vi "Configure FFT Measurement Trigger.vi"(4 "Trigger Timeout (1.0)":dbl=1.0 format="%^.3e", 5 "Offset (0.0)":dbl format="%^.3e", 6 "Threshold (-30.0)":dbl=-30.0 format="%^.3e", 7 "Slope (Rising)":i32(ring) items=["Rising", "Falling"], 8 "error in (no error)":errorcluster, 9 "Source (\"Free Run\")":string="Free Run", 10 "Instance (1)":i32=1, 11 "VISA resource name":refnum<visa-resource-name>) -> (0 "error out":errorcluster, 3 "VISA resource name out":refnum<visa-resource-name>)   [LabVIEW 2020, in "Rohde&Schwarz CMXP GPRF.lvlib"]
doc: "Defines the trigger parameters.\n\nAttributes:\nRSCMXPGPRF_ATTR_FFT_MEASUREMENT_TRIGGER_SOURCE\nRSCMXPGPRF_ATTR_FFT_MEASUREMENT_TRIGGER_SLOPE\nRSCMXPGPRF_ATTR_FFT_MEASUREMENT_TRIGGER_THRESHOLD\nRSCMXPGPRF_ATTR_FFT_MEASUREMENT_TRIGGER_OFFSET\nRSCMXPGPRF_ATTR_FFT_MEASUREMENT_TRIGGER_TIMEOUT\n\nRemote-control commands:\nTRIGger:GPRF:MEAS<i>:FFTSanalyzer:SOURce\nTRIGger:GPRF:MEAS<i>:FFTSanalyzer:SLOPe\nTRIGger:GPRF:MEAS<i>:FFTSanalyzer:THReshold\nTRIGger:GPRF:MEAS<i>:FFTSanalyzer:OFFSet\nTRIGger:GPRF:MEAS<i>:FFTSanalyzer:TOUT"
uses:
  <instrlib>/Rohde&Schwarz CMXP GPRF/Rohde&Schwarz CMXP GPRF.lvlib
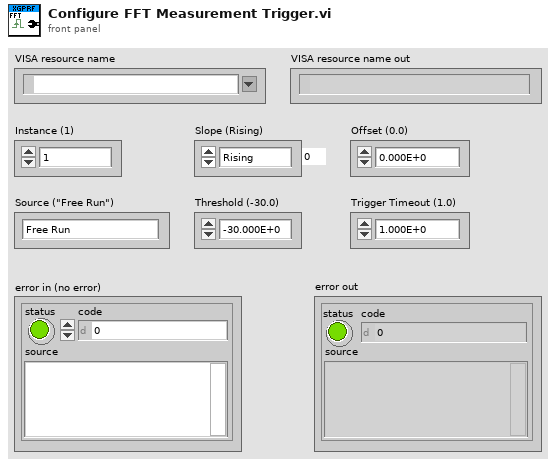
[diagram p1: front panel]
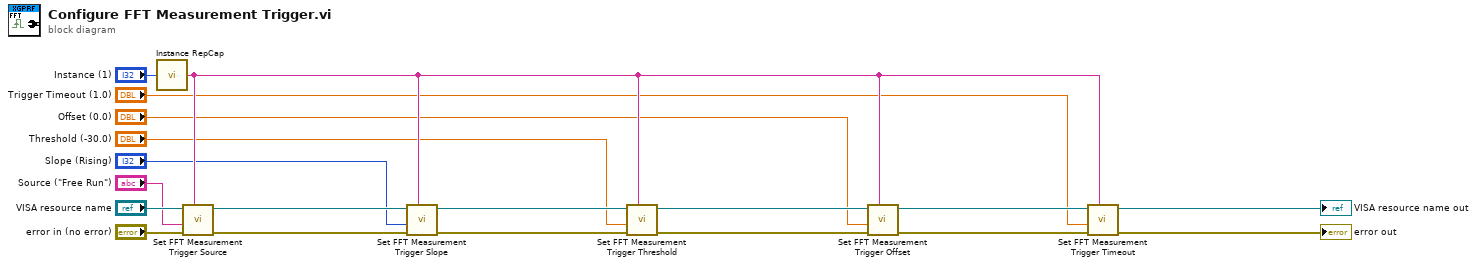
[diagram p0: block diagram]
diagram:
  n1 = call <instrlib>:"Instance RepCap.vi"("Instance in"="Instance (1)") -> ("Instance out"=w12:string)
  n2 = call "Set FFT Measurement Trigger Source"("Repeated Capabilities"=w12, "error in (no error)"="error in (no error)", "FFT Measurement Trigger Source ()"="Source (\"Free Run\")", "instrument handle"="VISA resource name") -> ("error out"=w16:errorcluster, "instrument handle out"=w15:refnum<visa-resource-name>)  [unwired: 6 in]
  n3 = call "Set FFT Measurement Trigger Slope"("Repeated Capabilities"=w12, "error in (no error)"=w16, "FFT Measurement Trigger Slope (0 - Rising)"="Slope (Rising)", "instrument handle"=w15) -> ("error out"=w14:errorcluster, "instrument handle out"=w13:refnum<visa-resource-name>)  [unwired: 6 in]
  n4 = call "Set FFT Measurement Trigger Threshold"("Repeated Capabilities"=w12, "error in (no error)"=w14, "FFT Measurement Trigger Threshold (0.0)"="Threshold (-30.0)", "instrument handle"=w13) -> ("error out"=w11:errorcluster, "instrument handle out"=w10:refnum<visa-resource-name>)  [unwired: 6 in]
  n5 = call "Set FFT Measurement Trigger Offset"("Repeated Capabilities"=w12, "error in (no error)"=w11, "FFT Measurement Trigger Offset (0.0)"="Offset (0.0)", "instrument handle"=w10) -> ("error out"=w9:errorcluster, "instrument handle out"=w8:refnum<visa-resource-name>)  [unwired: 6 in]
  n6 = call "Set FFT Measurement Trigger Timeout"("Repeated Capabilities"=w12, "error in (no error)"=w9, "FFT Measurement Trigger Timeout (0.0)"="Trigger Timeout (1.0)", "instrument handle"=w8) -> ("error out"=→"error out":errorcluster, "instrument handle out"=→"VISA resource name out":refnum<visa-resource-name>)  [unwired: 6 in]
